vi "MyDiscreteTF.vi"(5 "Denominator":fxp<+/-,32,10>[](array[numeric])=[0.0, 0.0, 0.0, 0.0, 0.0, 0.0, 0.0, 0.0], 7 "Numerator":fxp<+/-,32,10>[](array[numeric])=[0.0, 0.0, 0.0, 0.0, 0.0, 0.0, 0.0, 0.0], 9 "reset":bool, 10 "Input x(k)":fxp<+/-,32,10>, 11 "Order":i16) -> (2 "output":fxp<+/-,32,10>)   [LabVIEW 2011]
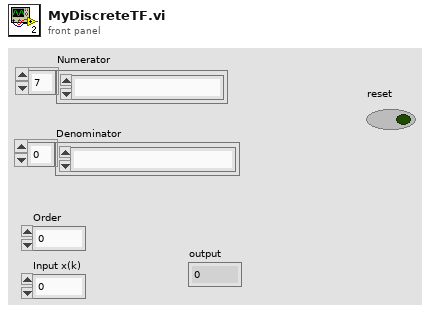
[diagram p1: front panel]
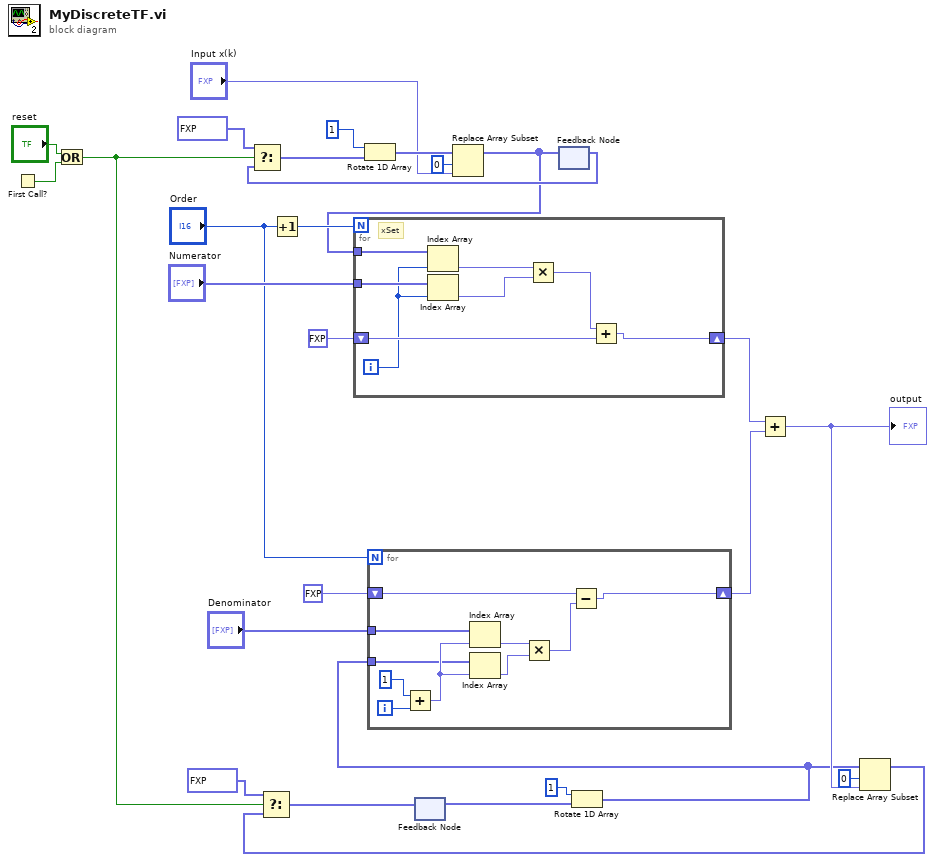
[diagram p0: block diagram]
diagram:
  n1 = First Call?() -> (First Call?: T/F=w18:bool)
  n2 = Or(x="reset", y=w18) -> (x .or. y?=w16:bool)
  n3 = Increment(x="Order") -> (x+1=w6:i16)
  n4 = feedback #1() -> (w3:fxp<+/-,64,32>[])  [unwired: 1 in]
  n5 = feedback #2() -> (w2:fxp<+/-,64,32>[])  [unwired: 1 in]
  n6 = Select(t=fxp<+/-,64,32>[] [0.0, 0.0, 0.0, 0.0, 0.0, 0.0, 0.0, 0.0], s=w16, f=w2) -> (s? t:f=w17:fxp<+/-,64,32>[])
  n7 = Rotate 1D Array(1:w17, 2:1 ("n")) -> (0:w24:fxp<+/-,64,32>[])
  n8 = Replace Array Subset(array=w24, new element="Input x(k)", index=0) -> (w1:fxp<+/-,64,32>[])
  n9 = for {
    N: w6 -> [_]
    tunnel: "Numerator" -> [w35]
    shift-right: [w33] -> w22
    shift-left: fxp<+/-,64,32> 0.0 ("Input x(k)") -> [w34]
    tunnel: w1 -> [w30]
    i -> [w28]
    # "xSet"
    n10 = Index Array(array=w30, index=w28) -> (element=w29:fxp<+/-,64,32>)
    n11 = Index Array(array=w35, index=w28) -> (element=w31:fxp<+/-,32,10>)
    n12 = Multiply(x=w29, y=w31) -> (x*y=w32:fxp<+/-,64,32>)
    n13 = Add(x=w32, y=w34) -> (x+y=w33:fxp<+/-,64,32>)
  }
  n14 = feedback-in #2(w1) -> ()
  n15 = Rotate 1D Array(1:w3, 2:1 ("n")) -> (0:w5:fxp<+/-,64,32>[])
  n16 = for {
    N: "Order" -> [_]
    tunnel: "Denominator" -> [w43]
    shift-right: [w36] -> w8
    shift-left: fxp<+/-,64,32> 0.0 ("Input x(k)") -> [w40]
    tunnel: w5 -> [w38]
    i -> [w45]
    n17 = Add(x=1, y=w45) -> (x+y=w42:fxp<+/-,64,32>)
    n18 = Index Array(array=w43, index=w42) -> (element=w41:fxp<+/-,32,10>)
    n19 = Index Array(array=w38, index=w42) -> (element=w39:fxp<+/-,64,32>)
    n20 = Multiply(x=w41, y=w39) -> (x*y=w37:fxp<+/-,64,32>)
    n21 = Subtract(x=w40, y=w37) -> (x-y=w36:fxp<+/-,64,32>)
  }
  n22 = Add(x=w22, y=w8) -> (x+y=w21:fxp<+/-,64,32>)
  "output" <- w21
  n23 = Replace Array Subset(array=w5, new element=w21, index=0) -> (w11:fxp<+/-,64,32>[])
  n24 = Select(t=fxp<+/-,64,32>[] [0.0, 0.0, 0.0, 0.0, 0.0, 0.0, 0.0, 0.0], s=w16, f=w11) -> (s? t:f=w4:fxp<+/-,64,32>[])
  n25 = feedback-in #1(w4) -> ()
